vi "CameraXY2projectorXY.vi"(9 "Linear Transformation Description":T1 {"mean error\n(projector pixels)" format="%0.2f"}, 11 "Camera Point":cluster{"X":sgl, "Y":sgl} {"Y" format="%.2f"; "X" format="%.2f"}) -> (3 "Projector Point":cluster{"X":sgl, "Y":sgl} {"Y" format="%.2f"; "X" format="%.2f"})   [LabVIEW 2019]
uses:
  LinearTransformationDescriptionCluster.ctl
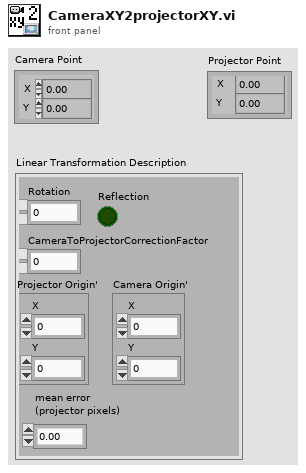
[diagram p1: front panel]
types:
  T1 = typedef "LinearTransformationDescriptionCluster.ctl" = cluster{"Rotation":sgl, "Reflection":bool, "CameraToProjectorCorrectionFactor":dbl, "Projector Origin'":cluster{"X":dbl, "Y":dbl}, "Camera Origin'":cluster{"X":dbl, "Y":dbl}, "mean error\n(projector pixels)":dbl}
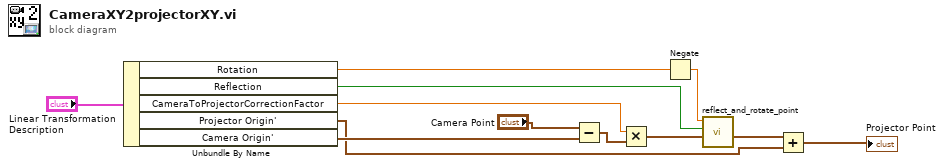
[diagram p0: block diagram]
diagram:
  n1 = Unbundle By Name("Linear Transformation Description") -> ("Rotation"=w6:sgl, "Reflection"=w5:bool, "CameraToProjectorCorrectionFactor"=w3:dbl, "Projector Origin'"=w1:cluster{"X":dbl, "Y":dbl}, "Camera Origin'"=w4:cluster{"X":dbl, "Y":dbl})
  n2 = Subtract(x="Camera Point", y=w4) -> (x-y=w2:cluster{"X":dbl, "Y":dbl})
  n3 = Multiply(x=w3, y=w2) -> (x*y=w11:cluster{"X":dbl, "Y":dbl})
  n4 = Negate(x=w6) -> (-x=w8:sgl)
  n5 = call "reflect_and_rotate_point.vi"("Point"=w11, "reflect about the x axis?"=w5, "rotation angle (radians)"=w8) -> ("transformed point"=w10:cluster{"X":sgl, "Y":sgl})  [unwired: 8 in]
  n6 = Add(x=w10, y=w1) -> (x+y=→"Projector Point":cluster{"X":dbl, "Y":dbl})
